vi "BGScriptGenerator.vi"(8 "Cycle time\n(ms)":i32=3 min=0 step=1, 9 "# Frames":i32=1000 min=0 step=1, 10 "BIN":u16(ring)=2 items=["1x1", "2x2", "4x4"], 11 "MODE":u16(ring) items=["Normal", "DIF"]) -> (0 "Duration (ms)":i32, 3 "BG Script":string)   [LabVIEW 2018]
panel:
  out "Wait":i32
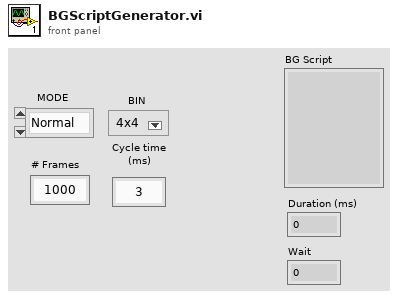
[diagram p1: front panel]
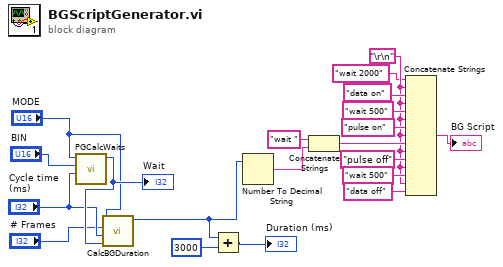
[diagram p0: block diagram]
diagram:
  w5 = "\r\n"
  n1 = call "PGCalcWaits.vi"("Cycle time\n(ms)"="Cycle time\n(ms)", "BIN"="BIN", "MODE"="MODE") -> ("Wait"=w13:i32)  [unwired: 8 in]
  "Wait" <- w13
  n2 = call "CalcBGDuration.vi"("Wait"=w13, "Cycle time\n(ms)"="Cycle time\n(ms)", "# Frames"="# Frames", "MODE"="MODE") -> ("Duration (ms)"=w3:i32)  [unwired: 7 in]
  n3 = Add(x=w3, y=3000) -> (x+y=→"Duration (ms)":i32)
  n4 = Number To Decimal String(number=w3) -> (decimal integer string=w9:string)  [unwired: 1 in]
  n5 = Concatenate Strings("wait " ("string"), w9) -> (w14:string)
  n6 = Concatenate Strings("wait 2000" ("string"), w5, "data on" ("string"), w5, "wait 500" ("string"), w5, "pulse on" ("string"), w5, w14, w5, "pulse off" ("string"), w5, "wait 500" ("string"), w5, "data off" ("string")) -> (→"BG Script":string)
